vi "Write_MessageHandler_MessageNb.vi"(8 "error in (no error)":errorcluster, 10 "Message number":u32, 11 "MessageHandler in":refnum<class "MessageHandler.lvclass">) -> (0 "error out":errorcluster, 3 "MessageHandler out":refnum<class "MessageHandler.lvclass">)   [LabVIEW 2013, in "MessageHandler.lvclass"]
uses:
  MessageHandler.lvclass
  MessageHandler.lvclass/MessageHandler.ctl
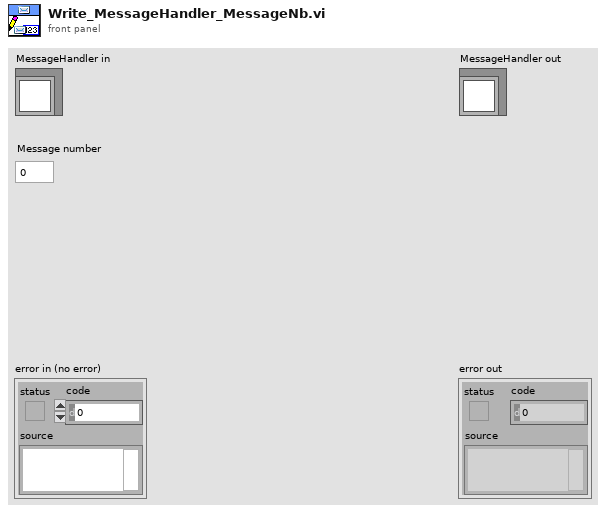
[diagram p1: front panel]
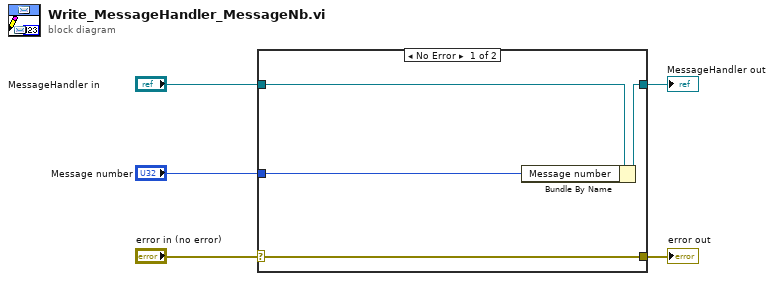
[diagram p0: block diagram]
diagram:
  n1 = case shown="No Error" "error in (no error)" {
    selector: "error in (no error)" -> [w9 w10]
    tunnel: [w9 w10] -> w4
    tunnel: [w7 w11] -> w2
    tunnel: "MessageHandler in" -> [w8 w11]
    tunnel: "Message number" -> [w6 _]
    frame No Error {
      n2 = Bundle By Name(cluster=w8, "Message number"=w6) -> (w7:refnum<class "MessageHandler.lvclass">)
    }
    frame Error {
    }
  }
  "error out" <- w4
  "MessageHandler out" <- w2
